vi "APS absolute arc move 3pe.vi"(0 "Dimension":i32, 1 "Max_Arc_Speed":i32, 5 "Axis_ID_Array":i32, 7 "Pass_Pos_Array":i32, 9 "End_Pos_Array":i32, 11 "error in (no error)":errorcluster caption="错误输入（无错误）") -> (4 "function return":i32, 6 "Axis_ID_Array out":i32, 8 "Pass_Pos_Array out":i32, 10 "End_Pos_Array out":i32, 15 "error out":errorcluster caption="错误输出")   [LabVIEW 2017, in "APS168.lvlib"]
doc: "I32 FNTYPE APS_absolute_arc_move_3pe(I32 Dimension, I32 *Axis_ID_Array, I32 *Pass_Pos_Array, I32 *End_Pos_Array, I32 Max_Arc_Speed );"
uses:
  APS168.lvlib
  APS168.dll
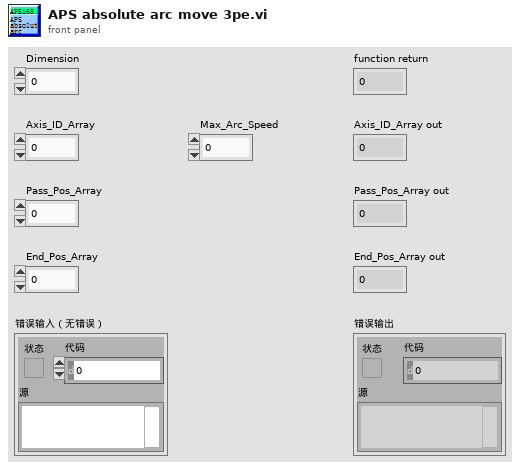
[diagram p1: front panel]
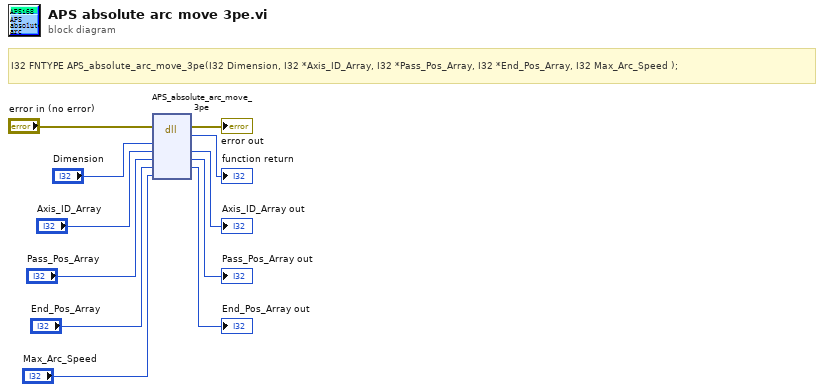
[diagram p0: block diagram]
diagram:
  # "I32 FNTYPE APS_absolute_arc_move_3pe(I32 Dimension, I32 *Axis_ID_Array, I32 *Pass_Pos_Array, I32 *End_Pos_Array, I32 Max_Arc_Speed );"
  n1 = dll-call lib="PTH2Gabs E迈治LV范例testSubVIsADLINKMotion204cAPS168.*" fn="APS_absolute_arc_move_3pe"(error in="error in (no error)", "Dimension"="Dimension", "Axis_ID_Array"="Axis_ID_Array", "Pass_Pos_Array"="Pass_Pos_Array", "End_Pos_Array"="End_Pos_Array", "Max_Arc_Speed"="Max_Arc_Speed") -> (error out=→"error out":errorcluster, →"function return":i32, "Axis_ID_Array"=→"Axis_ID_Array out":i32, "Pass_Pos_Array"=→"Pass_Pos_Array out":i32, "End_Pos_Array"=→"End_Pos_Array out":i32)  [unwired: 4 in, 1 out]
